vi "Robot Global Data.vi"() -> ()   [LabVIEW 2020]
doc: "This global VI can contain as many global variables as you need. Place a control on the panel, give it a good name. To read or write to it from a VI, drag the icon to the diagram of that VI. You can also drag from the project. Click on the node to change which global you access. You shouldn't have multiple locations writing to a global or it will cause a race-condition."
uses:
  <vilib>/Rock Robotics/WPI/Camera/WPI_CameraImageSize.ctl
  <vilib>/Rock Robotics/WPI/DriverStation/WPI_DriverStationRobotMode2.ctl
panel:
  in  "OC_Eject":bool
  in  "OC_Shoot Off":bool
  in  "Backup":bool
  in  "DC_Backup":bool
  in  "OC_Align VY":bool
  out "Auto Type":i8
  in  "OC_Change Lights":bool
  in  "Arduino":bool
  in  "Change Lights":bool
  in  "Robot Lights":i8
  out "D Set Lights":i8
  out "Desired Dist":dbl
  in  "OC_Tee Pot Man":bool
  in  "Fly_Adjust":bool
  out "Target Dist":dbl
  out "Lime Y Angle":dbl
  out "Set Y Offset":dbl
  out "LED Mode":i8
  out "Cam Mode":i8
  in  "Centering":bool
  in  "VY Align":bool
  in  "VX Align":bool
  out "Lime Y":dbl
  in  "LED Reset":bool
  in  "DC_Shoot":bool
  in  "OC_ Flywheel Off":bool
  in  "OC_ Flywheel On":bool
  in  "Finish":bool
  out "DC Tee Pwr":dbl
  out "Auto Tee Pwr":dbl
  out "OC_Tee Pwr":dbl
  in  "OC_Chaos":bool
  out "Raw Tee Pot":dbl
  in  "OC_ Tee Normal Power":bool
  in  "OC_ TB Override":bool
  in  "Tee Lo Power":bool
  in  "OC_Climb Off":bool
  in  "OC_Climb On":bool
  in  "Flywheel On":bool
  in  "Intake On":bool
  in  "OC_ Intake On":bool
  out "Tee Speed":dbl format="%.2f"
  out "TBar R":dbl
  out "TBar L":dbl
  in  "OC_Align VX":bool
  in  "OC_ Hook":bool
  in  "OC_ Tee":bool
  in  "OC_U":bool
  in  "TB_Out":bool
  in  "Cargo":bool
  out "Intake Pwr":dbl
  in  "Tee-Out":bool
  out "Tee Pwr":dbl
  out "Desired Tee_Pot":dbl
  out "Tee_Pot":dbl
  in  "Climb On":bool
  out "Carriage Piston Position":dbl
  in  "Carriage Down":bool
  in  "Carriage Up":bool
  in  "OC_ Long":bool
  in  "Long Shot":bool
  in  "Fender High":bool
  in  "Fender Low":bool
  in  "Carriage Pos":T1(ring)
  in  "OC_ High":bool
  in  "OC_Low":bool
  out "Desired Speed":dbl
  out "Flywheel Speed":dbl
  out "Flywheel Power":dbl
  in  "OC_Shoot":bool
  in  "LS On 2":bool
  out "Climb Piston Position":dbl
  in  "OC_TB Out":bool
  in  "OC_TB In":bool
  out "TB Power":dbl
  out "Fal Enc Reset":dbl format="%.2f"
  out "Falcon Encoder":dbl format="%.2f"
  out "Fal Enc Raw":dbl format="%.2f"
  out "Talon SRX 2":dbl
  in  "Victor SP":bool
  out "Falcon":dbl
  out "Dash Y":dbl
  out "Score":i8
  in  "DC_Forward":bool
  in  "DC_Reverse":bool
  in  "Lo LS":bool
  in  "Hi LS":bool
  in  "LS On":bool
  in  "DC_Halo On":bool
  in  "Halo On":bool
  in  "OC_Tee":bool
  out "Talon SRX 1":dbl(knob) scale=-1.0..1.0
  in  "OC_Cargo":bool
  in  "OC_LA_Reset":bool
  in  "OC_Rumble":bool
  out "Photo LS Num":dbl
  out "Drv Input 2":dbl
  out "Drv Input 1":dbl
  in  "OC_Piston Up":bool
  in  "DC_Auto TS":bool
  in  "DC_A Align TS":bool
  in  "DC_D_Enc-R":bool
  in  "DC_Normal":bool
  in  "DC_Precision":bool
  out "A Drv-R":dbl
  out "A Drv-L":dbl
  in  "LED 9":bool
  in  "LED 8":bool
  in  "LED 7":bool
  in  "LED 6":bool
  in  "LED 5":bool
  in  "LED 3":bool
  in  "LED 4":bool
  in  "LED 1":bool
  in  "LED 2":bool
  out "O_Encoder":dbl(knob) scale=-90.0..270.0
  out "Sonar":dbl
  in  "G Offset":dbl
  out "G Cal":dbl
  in  "Gyro Reset":bool
  in  "Photo LS On":bool
  in  "O_Enc-R":bool
  in  "Piston Up":bool
  out "Distance":dbl
  out "Y":dbl
  out "Score":dbl
  out "X":dbl
  out "Z-Axis":dbl format="%.2f"
  out "Y-Axis":dbl format="%.2f"
  out "X-Axis":dbl format="%.2f"
  out "Gyro":dbl
  out "Drift Cal":dbl
  out "Turn Cal":dbl
  in  "Locked On":bool
  in  "Tracking":bool
  in  "A Drv":bool
  in  "A Exit":bool
  in  "Drv Spd Av":dbl(knob) scale=-30.0..30.0
  out "Drv Dist Av":dbl
  out "Drv Dist R":dbl format="%.2f"
  out "Drv Spd R":dbl format="%.2f"
  out "Drv Dist L":dbl format="%.2f"
  out "Drv Spd L":dbl format="%.2f"
  in  "D_Enc-R":bool
  in  "Reverse":bool
  in  "Precision":bool
  in  "Drv-R-Out":dbl(knob) scale=-1.0..1.0
  in  "Drv-L-Out":dbl(knob) scale=1.0..-1.0
  out "Drive":string(combo)="Cheesy"
  out "D_Buttons":T2
  out "O2_Buttons":T2
  out "O2_Axis":T3
  out "O1_Axis":T3
  out "D_Axis":T3
  out "O1_Buttons":T2
  out "O2_POV":dbl
  out "O1_POV":dbl
  out "D_POV":dbl
  in  "Rumble":bool
  in  "Rumble Time":dbl
  out "Current Light":string(combo)="Select"
  out "Light Select":i8
  out "O_Controller":string(combo)="XBox"
  out "D_Controller":string(combo)="XBox"
  in  "U Button":bool
  in  "Lime Cam":bool
  out "VP Select":string(combo)="XBox"
  in  "Dash In View":bool
  in  "Lime In View":bool
  in  "VP In View":bool
  out "VP X":dbl(knob) scale=-150.0..150.0
  out "Lime X":dbl
  in  "Snapshot":bool
  out "Dash X":dbl
  out "Stream":i8
  out "CamMode":i8
  out "LedMode":i8
  out "Count":dbl
  out "V06":dbl
  out "V08":dbl
  out "V00":dbl
  out "V11":dbl
  out "Key Pressed":T4(array[ring])
  out "Key Enum":i16
  out "V10":dbl
  out "V09":dbl
  out "Auto TS":i8
  out "Dash Select":i8
  out "V07":dbl
  out "V05":dbl
  out "V04":dbl
  out "V03":dbl
  out "V02":dbl
  out "V01":dbl
  out "Game Data":string
  out "Tele Time":dbl
  out "Auto Time":dbl
  in  "Robot Mode":T5
  in  "image size":T6=enum."320x240"
  in  "Enable Vision":bool
  # "External Controls"
  # "Dashboard"
  # "Vision Processing"
  # "User Controls"
  # "Controller Variables"
  # "Dash Array"
  # "Operator Functions"
  # "Driver Functions"
  # "Driver Control Variables"
  # "Operator Control Variables"
  # "Diagnostics"
  # "^^^Replace with Select?"
  # "Vision Tracking"
  # "Accelerometer"
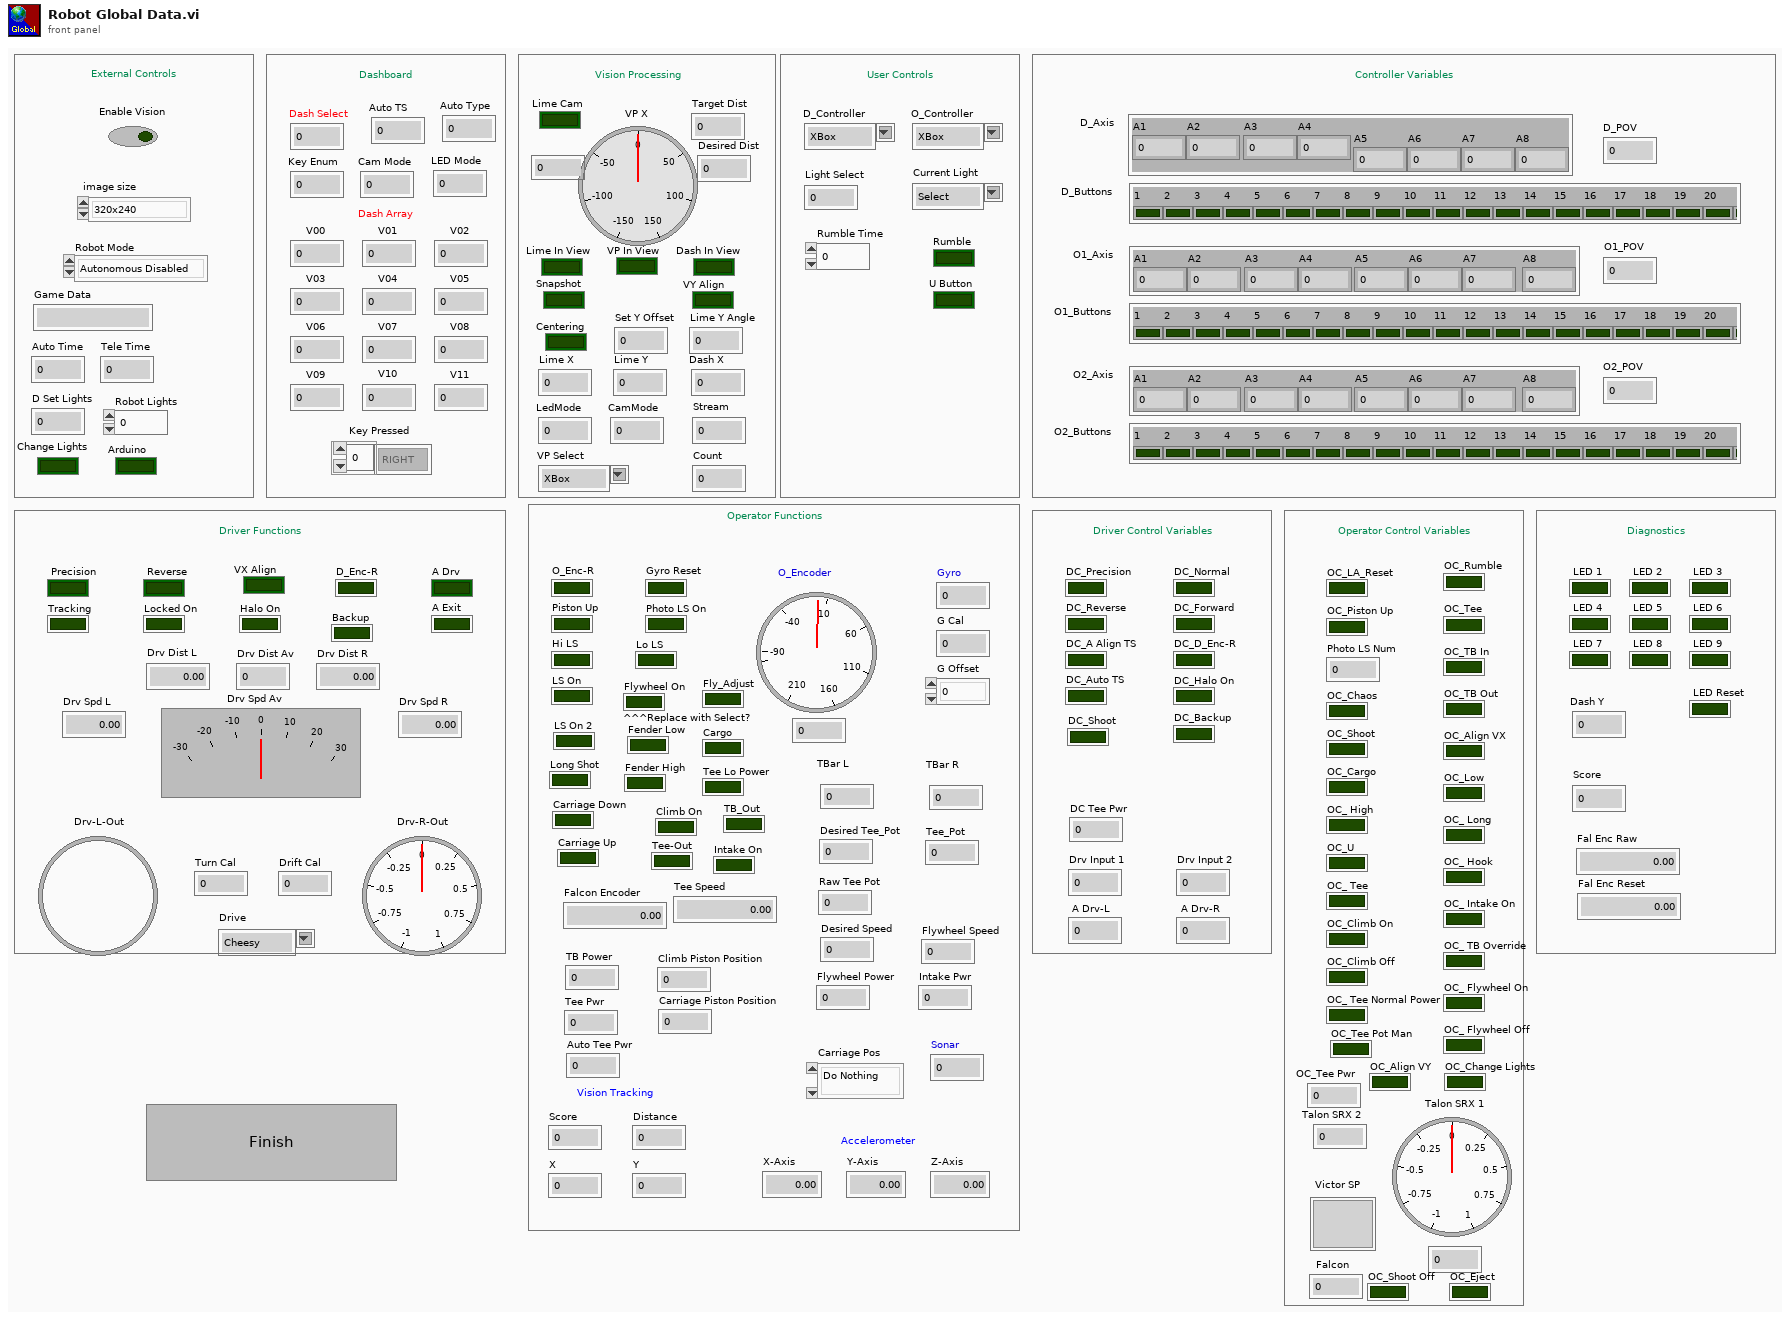
[diagram p1: front panel]
types:
  T1 = enum16{"Do Nothing", "Cargo", "Low", "High", "Long Shot", "U", "Hook", "Tee", "Eject"}
  T2 = cluster{"1":bool, "2":bool, "3":bool, "4":bool, "5":bool, "6":bool, "7":bool, "8":bool, "9":bool, "10":bool, "11":bool, "12":bool, "13":bool, "14":bool, "15":bool, "16":bool, "17":bool, "18":bool, "19":bool, "20":bool, "21":bool, "22":bool, "23":bool, "24":bool, "25":bool, "26":bool, "27":bool, "28":bool, "29":bool, "30":bool, "31":bool, "32":bool, "33":bool, "34":bool, "35":bool, "36":bool, "37":bool, "38":bool, "39":bool, "40":bool, "41":bool, "42":bool, "43":bool, "44":bool, "45":bool, "46":bool, "47":bool, "48":bool, "49":bool, "50":bool}
  T3 = cluster{"A1":dbl, "A2":dbl, "A3":dbl, "A4":dbl, "A5":dbl, "A6":dbl, "A7":dbl, "A8":dbl}
  T4 = enum16{"0", "1", "2", "3", "4", "5", "6", "7", "8", "9", "A", "B", "C", "D", "E", "F", "G", "H", "I", "J", "K", "L", "M", "N", "O", "P", "Q", "R", "S", "T", "U", "V", "W", "X", "Y", "Z", "F1", "F2", "F3", "F4", "F5", "F6", "F7", "F8", "F9", "F10", "F11", "F12", "F13", "F14", "F15", "ADD", "BACK", "BACKSLASH", "CAPITAL", "COMMA", "DECIMAL", "DELETE", "DIVIDE", "DOWN", "END", "EQUALS", "ESCAPE", "GRAVE (`)", "HOME", "INSERT", "LBRACKET", "LCONTROL", "LEFT", "L ALT", "LSHIFT", "LWIN", "MINUS", "MULTIPLY", "NEXT", "NUMLOCK", "NUMPAD_0", "NUMPAD_1", "NUMPAD_2", "NUMPAD_3", "NUMPAD_4", "NUMPAD_5", "NUMPAD_6", "NUMPAD_7", "NUMPAD_8", "NUMPAD_9", "PAUSE", "PERIOD", "PRIOR (PG UP)", "RBRACKET", "RCONTROL", "RETURN", "RIGHT", "R ALT", "RSHIFT", "RWIN", "SCROLL", "SEMICOLON", "SLASH", "SPACE", "SUBTRACT", "TAB", "UP", "ENTER (num pad)", "' (quote)"}[]
  T5 = typedef "WPI_DriverStationRobotMode2.ctl" = enum16{"Autonomous Disabled", "Autonomous Enabled", "Teleop Disabled", "Teleop Enabled", "Disconnected", "Finish", "Test Disabled", "Test Enabled", "Emergency Stopped"}
  T6 = typedef "WPI_CameraImageSize.ctl" = enum16{"640x480", "320x240", "160x120", "Custom"}
diagram:
